vi "FocusItemInListbox.vi"(8 "error in (no error)":errorcluster, 10 "patientID":string, 11 "ListBox in":refnum<vi>) -> (0 "error out":errorcluster)   [LabVIEW 2013, in "main.lvlib"]
uses:
  main.lvlib
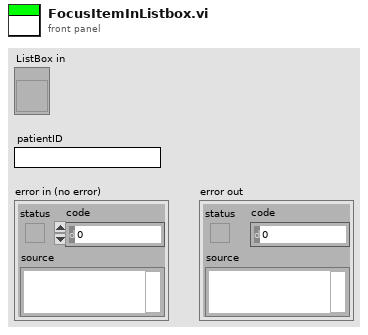
[diagram p1: front panel]
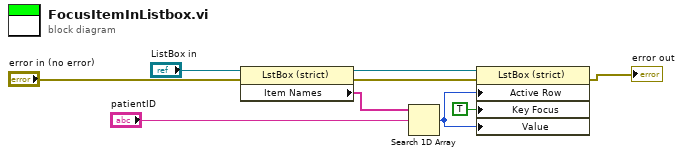
[diagram p0: block diagram]
diagram:
  n1 = property class="LstBox (strict)"(reference="ListBox in", error in="error in (no error)") -> (reference out=w3:refnum<vi>, error out=w4:errorcluster, "Item Names"=w6:string[])
  n2 = Search 1D Array(1D array=w6, element="patientID") -> (index of element=w7:i32)  [unwired: 1 in]
  n3 = property class="LstBox (strict)"(reference=w3, error in=w4, "Active Row"=w7, "Key Focus"=TRUE, "Value"=w7) -> (error out=→"error out":errorcluster)  [unwired: 1 out]
